vi "ZK_GetPosition.vi"(0 "Image Out 2":T1, 11 "error in":errorcluster) -> (6 "Calibrated Matches 2":T2(array[cluster]), 15 "error out":errorcluster)   [LabVIEW 2018]
uses:
  <vilib>/vision/Image Controls.llb/IMAQ Image.ctl
  <vilib>/vision/NI_Vision_Development_Module.lvlib
panel:
  out "Array":path[](array[path])
  out "Image Out":T1(plugin-control)
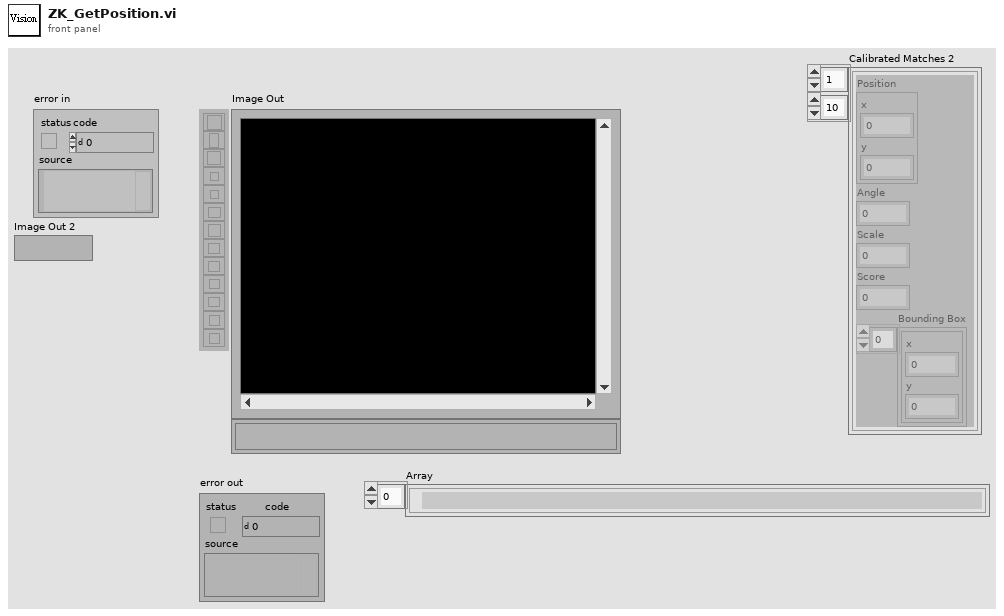
[diagram p1: front panel]
types:
  T1 = typedef "IMAQ Image.ctl" = refnum<image>
  T2 = cluster{"Position":cluster{"x":sgl, "y":sgl}, "Angle":sgl, "Scale":sgl, "Score":sgl, "Bounding Box":cluster{"x":sgl, "y":sgl}[]}[][]
  T3 = cluster{"Global Rectangle":i32[], "Contours":cluster{"ID":enum32{"External", "Internal"}, "Type":u32, "Coordinates":i32[]}[]}
  T4 = typedef "Image Type" = u32
  T5 = cluster{"Position":cluster{"x":sgl, "y":sgl}, "Angle":sgl, "Scale":sgl, "Score":sgl, "Bounding Box":cluster{"x":sgl, "y":sgl}[]}[]
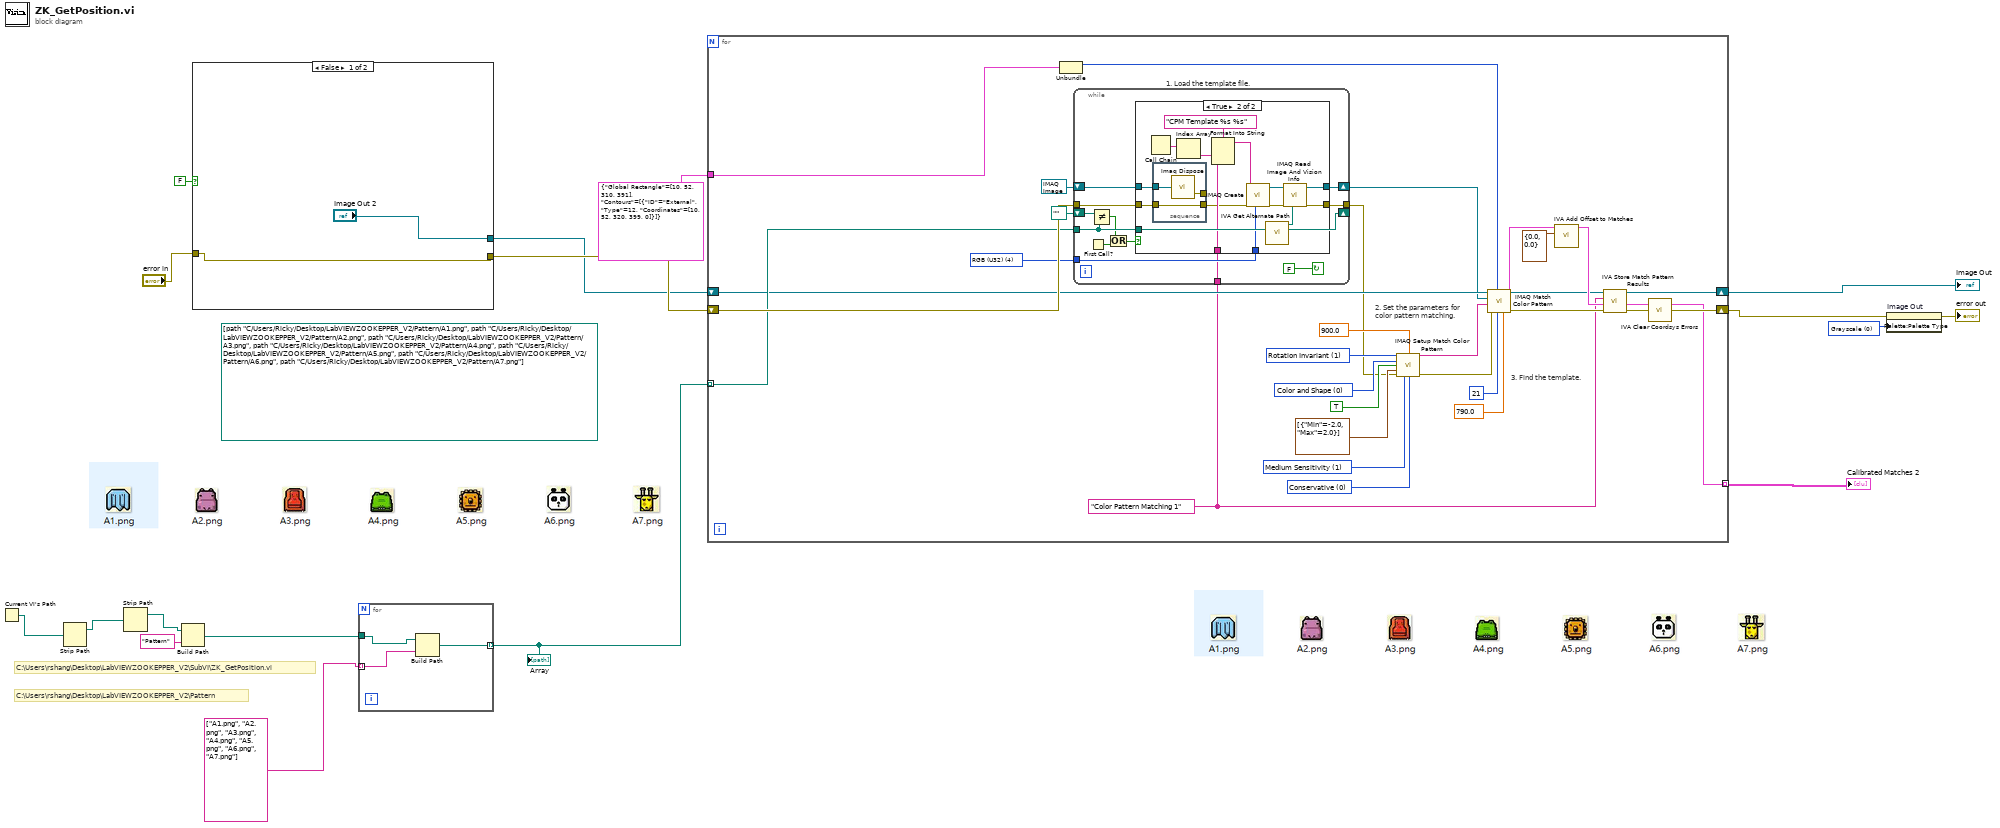
[diagram p0: block diagram]
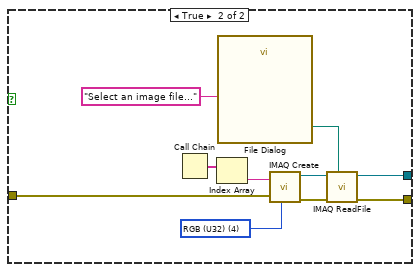
[diagram p2: hidden frame]
diagram:
  (unwired) path[] [path "C:/Users/Ricky/Desktop/LabVIEWZOOKEPPER_V2/Pattern/A1.png", path "C:/Users/Ricky/Desktop/LabVIEWZOOKEPPER_V2/Pattern/A2.png", path "C:/Users/Ricky/Desktop/LabVIEWZOOKEPPER_V2/Pattern/A3.png", path "C:/Users/Ricky/Desktop/LabVIEWZOOKEPPER_V2/Pattern/A4.png", path "C:/Users/Ricky/Desktop/LabVIEWZOOKEPPER_V2/Pattern/A5.png", path "C:/Users/Ricky/Desktop/LabVIEWZOOKEPPER_V2/Pattern/A6.png", path "C:/Users/Ricky/Desktop/LabVIEWZOOKEPPER_V2/Pattern/A7.png"] ("Array")
  w11 = u32 0 items=["Grayscale", "Binary", "Gradient", "Rainbow", "Temperature", "User Defined", "Binary 16 Bit", "Gradient 16 Bit", "Rainbow 16 Bit", "Temperature 16 Bit", "User Defined 16 Bit"] ("Palette Type")
  # "C:\\Users\\rshang\\Desktop\\LabVIEWZOOKEPPER_V2\\SubVI\\ZK_GetPosition.vi"
  # "C:\\Users\\rshang\\Desktop\\LabVIEWZOOKEPPER_V2\\Pattern"
  n1 = Current VI's Path() -> (path=w7:path)
  n2 = Strip Path(path=w7) -> (stripped path=w6:path)  [unwired: 1 out]
  n3 = Strip Path(path=w6) -> (stripped path=w5:path)  [unwired: 1 out]
  n4 = Build Path(base path=w5, name or relative path="Pattern") -> (appended path=w3:path)
  n5 = case shown="False" FALSE {
    tunnel: [w18 w29] -> w17
    tunnel: ["Image Out 2" w21] -> w15
    tunnel: "error in" -> [w18 w20]
    frame False {
    }
    frame True {
      w22 = T4 4 items=["Grayscale (U8)", "Grayscale (I16)", "Grayscale (SGL)", "Complex (CSG)", "RGB (U32)", "HSL (U32)", "RGB (U64)", "Grayscale (U16)"] ("Image Type")
      n6 = Call Chain() -> (call chain=w26:string[])
      n7 = Index Array(array=w26) -> (element=w25:string)  [unwired: 1 in]
      n8 = call "File Dialog"("prompt"="Select an image file...") -> ("selected path"=w23:path)  [unwired: 6 in, 8 out]
      n9 = call "IMAQ Create"("Image Name"=w25, "Image Type"=w22, "error in (no error)"=w20) -> ("New Image"=w28:T1, "error out"=w27:errorcluster)  [unwired: 1 in, 1 out]
      n10 = call "IMAQ ReadFile"("File Path"=w23, "error in (no error)"=w27, "Image"=w28) -> ("error out"=w29:errorcluster, "Image Out"=w21:T1)  [unwired: 2 in, 5 out]
    }
  }
  n11 = for {
    tunnel: w3 -> [w32]
    tunnel: string[] ["A1.png", "A2.png", "A3.png", "A4.png", "A5.png", "A6.png", "A7.png"] -> [w31] mode=indexing
    tunnel: [w30] -> w1 mode=indexing
    n12 = Build Path(base path=w32, name or relative path=w31) -> (appended path=w30:path)
  }
  "Array" <- w1
  n13 = for {
    tunnel: w1 -> [w53] mode=indexing
    tunnel: T3 {"Global Rectangle"=[10, 52, 310, 391], "Contours"=[{"ID"=enum."External", "Type"=12, "Coordinates"=[10, 52, 320, 399, 0]}]} ("ROI Descriptor") -> [w49]
    shift-right: [w37] -> w14
    shift-left: w17 -> [w62]
    shift-right: [w36] -> w12
    shift-left: w15 -> [w46]
    tunnel: [w35] -> w10 mode=indexing
    w45 = "Color Pattern Matching 1" ("Step Name")
    w52 = T4 4 items=["Grayscale (U8)", "Grayscale (I16)", "Grayscale (SGL)", "Complex (CSG)", "RGB (U32)", "HSL (U32)", "RGB (U64)"] ("Image Type")
    w55 = u32 0 items=["Conservative", "Balance", "Aggressive", "Very Aggressive"] ("Search Strategy")
    w56 = u32 1 items=["Low Sensitivity", "Medium Sensitivity", "High Sensitivity"] ("Color Sensitivity")
    w58 = u32 0 items=["Color and Shape", "Color", "Shape"] ("Match Feature Mode")
    w59 = u32 1 items=["Shift Invariant", "Rotation Invariant"] ("Match Mode")
    # "2. Set the parameters for\ncolor pattern matching."
    # "3. Find the template."
    n14 = Unbundle(w49) -> ("Global Rectangle"=w41:i32[])  [unwired: 1 out]
    n15 = while "1. Load the template file." {
      shift-right: [w74] -> w40
      shift-left: T1 refnum ("Image Out") -> [w73]
      tunnel: [w71] -> w39
      tunnel: w62 -> [w70]
      tunnel: w53 -> [w66]
      tunnel: w52 -> [w69]
      tunnel: w45 -> [w68]
      shift-right: [w66] -> _
      shift-left: path "" ("File Path") -> [w67]
      stop <- FALSE continue-if-true
      n16 = First Call?() -> (First Call?: T/F=w65:bool)
      n17 = Not Equal?(x=w67, y=w66) -> (x != y?=w64:bool)
      n18 = Or(x=w64, y=w65) -> (x .or. y?=w63:bool)
      n19 = case shown="True" w63 {
        tunnel: [w76 w89] -> w74
        tunnel: w73 -> [w76 w81]
        tunnel: [w75 w86] -> w71
        tunnel: w70 -> [w75 w80]
        tunnel: w66 -> [_ w78]
        tunnel: w69 -> [_ w85]
        tunnel: w68 -> [_ w82]
        frame False {
        }
        frame True {
          n20 = Call Chain() -> (call chain=w84:string[])
          n21 = stacked-sequence {
            tunnel: w81 -> [w94]
            tunnel: w80 -> [w93]
            tunnel: [w93] -> w79
            tunnel: [w92] -> _
            frame #0 {
              n22 = call "Imaq Dispose"("Image"=w94) -> ("error out"=w92:errorcluster)  [unwired: 2 in, 3 out]
            }
          }
          n23 = Index Array(array=w84) -> (element=w83:string)  [unwired: 1 in]
          n24 = Format Into String(format string="CPM Template %s %s" ("Image Name"), w83, w82) -> (resulting string=w91:string)  [unwired: 2 in, 1 out]
          n25 = call "IMAQ Create"("Image Name"=w91, "Image Type"=w85, "error in (no error)"=w79) -> ("New Image"=w88:T1, "error out"=w87:errorcluster)  [unwired: 1 in, 1 out]
          n26 = call <vilib>:"IVA Get Alternate Path.vi"("Path In"=w78) -> ("Path Out"=w77:path)  [unwired: 10 out]
          n27 = call "IMAQ Read Image And Vision Info"("File Path"=w77, "error in (no error)"=w87, "Image"=w88) -> ("error out"=w86:errorcluster, "Image Out"=w89:T1)  [unwired: 1 in, 6 out]
        }
      }
    }
    n28 = call "IMAQ Setup Match Color Pattern"("Match Mode"=w59, "Color Score Weight"=sgl 900.0, "Match Feature Mode"=w58, "Subpixel Accuracy"=TRUE, "Rotation Angle Ranges (degrees)"=cluster{"Min":sgl, "Max":sgl}[] [{"Min"=-2.0, "Max"=2.0}], "error in (no error)"=w39, "Color Sensitivity"=w56, "Search Strategy"=w55) -> ("Match Color Pattern Setup Data"=w44:string, "error out"=w43:errorcluster)  [unwired: 1 in, 5 out]
    n29 = call "IMAQ Match Color Pattern"("Minimum Match Score"=sgl 790.0, "Number of Matches Requested"=21, "Optional Rectangle"=w41, "error in (no error)"=w43, "Match Color Pattern Setup Data"=w44, "Template Image"=w40, "Image"=w46) -> ("error out"=w47:errorcluster, "Matches"=w42:T5)  [unwired: 3 out]
    n30 = call <vilib>:"IVA Add Offset to Matches.vi"("Match Offset"=cluster{"X":sgl, "Y":sgl} {"X"=0.0, "Y"=0.0}, "Matches in"=w42) -> ("Matches out"=w48:T5)  [unwired: 9 out]
    n31 = call <vilib>:"IVA Store Match Pattern Results.vi"("error in (no error)"=w47, "Matches"=w48, "Step Name"=w45, "Image in"=w46) -> ("error out"=w38:errorcluster, "Calibrated Matches"=w35:T5, "Image dup"=w36:T1)  [unwired: 5 out]
    n32 = call <vilib>:"IVA Clear Coordsys Errors.vi"("error in (no error)"=w38) -> ("error out"=w37:errorcluster)  [unwired: 10 in]
  }
  "Image Out" <- w12
  "Calibrated Matches 2" <- w10
  n33 = property on="Image Out" class="ImageControl"(error in=w14, "Palette:Palette Type"=w11) -> (error out=→"error out":errorcluster)  [unwired: 1 in, 1 out]
